vi "Thread_dw.vi"(2 "에러 입력(에러 없음)":errorcluster, 3 "α":dbl, 4 "P":dbl) -> (0 "에러 출력":errorcluster, 1 "결과":dbl)   [LabVIEW 2020]
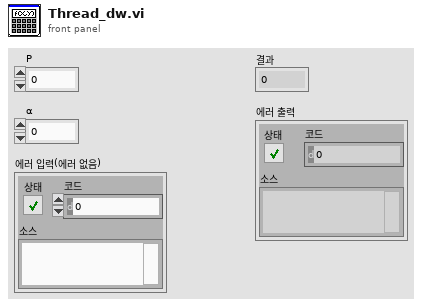
[diagram p1: front panel]
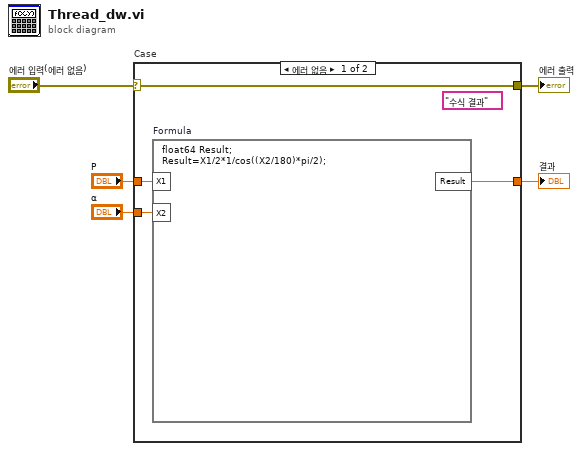
[diagram p0: block diagram]
diagram:
  n1 = case "Case" shown="에러 없음" "에러 입력(에러 없음)" {
    selector: "에러 입력(에러 없음)" -> [w6 w10]
    tunnel: [w7 _] -> w2
    tunnel: [w6 w10] -> w1
    tunnel: "P" -> [w9 _]
    tunnel: "α" -> [w8 _]
    frame No Error {
      (unwired) "수식 결과" ("Name Modifier")
      n2 = formula code="float64 Result;\nResult=X1/2*1/cos((X2/180)*pi/2);"("X1"=w9, "X2"=w8) -> ("Result"=w7:dbl)
    }
    frame Error {
    }
  }
  "결과" <- w2
  "에러 출력" <- w1
